vi "Parse Step Type.vi"(8 "error in (no error)":errorcluster, 9 "Sequence Context":refnum<class "Configuration.lvclass">, 10 "TestStand Result in":T2) -> (0 "error out":errorcluster, 2 "Step Type":T1=enum."String Value Test")   [LabVIEW 2020, in "Astemes_CSVReportPlugin.lvlib" / "TestStand Result Handler.lvclass"]
uses:
  TestStand Result Handler.lvclass
  Step Types.ctl
  Configuration/Configuration.lvclass
  TestStand Result.ctl
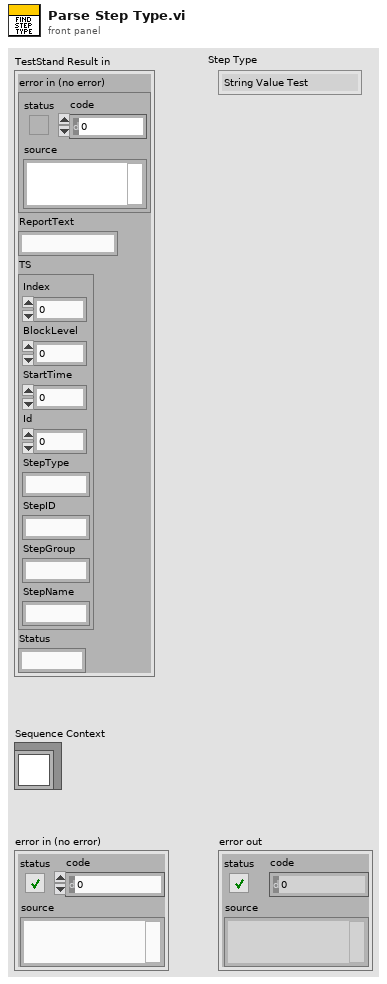
[diagram p1: front panel]
types:
  T1 = typedef "Astemes_CSVReportPlugin.lvlib/TestStand Result Handler.lvclass/Step Types.ctl" = enum16{"Unknown", "String Value Test", "Numeric Limit Test", "Action", "Flow Control"}
  T2 = typedef "Astemes_CSVReportPlugin.lvlib/TestStand Result Handler.lvclass/TestStand Result.ctl" = cluster{"error in (no error)":errorcluster, "ReportText":string, "TS":cluster{"Index":i32, "BlockLevel":i32, "StartTime":dbl, "Id":i32, "StepType":string, "StepID":string, "StepGroup":string, "StepName":string}, "Status":string}
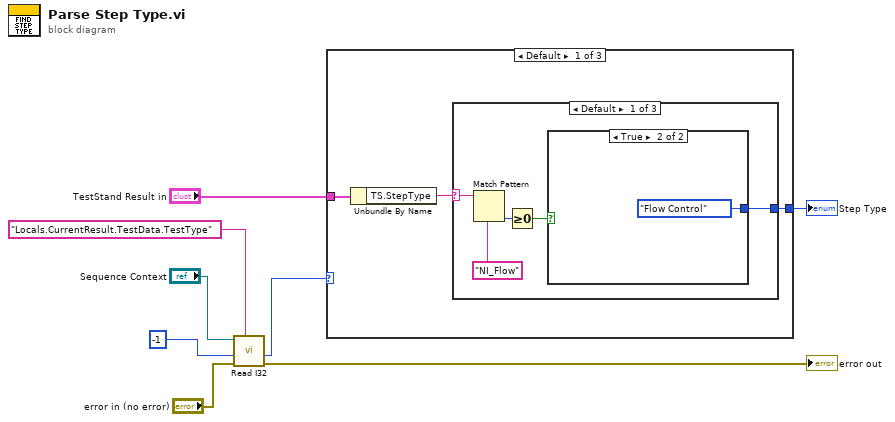
[diagram p0: block diagram]
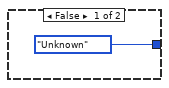
[diagram p2: hidden frame]
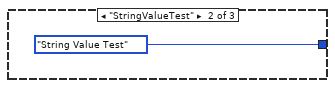
[diagram p3: hidden frame]
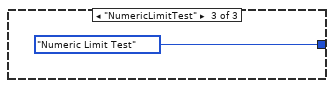
[diagram p4: hidden frame]
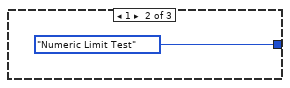
[diagram p5: hidden frame]
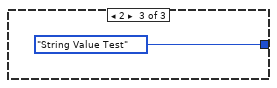
[diagram p6: hidden frame]
diagram:
  n1 = call-dynamic "Read I32.vi"("key"="Locals.CurrentResult.TestData.TestType", "error in (no error)"="error in (no error)", "default value"=-1, "Configuration In"="Sequence Context") -> ("error out"=→"error out":errorcluster, "value"=w2:i32)  [unwired: 5 in, 1 out]
  n2 = case shown="Default" w2 {
    tunnel: "TestStand Result in" -> [w11 _ _]
    tunnel: [w9 Step_Types."Numeric Limit Test" ("Step Type") Step_Types."String Value Test" ("Step Type")] -> w6
    frame Default {
      n3 = Unbundle By Name(w11) -> ("TS.StepType"=w10:string)
      n4 = case shown="Default" w10 {
        selector: w10 -> [w15 _ _]
        tunnel: [w16 Step_Types."String Value Test" ("Step Type") Step_Types."Numeric Limit Test" ("Step Type")] -> w9
        frame Default {
          n5 = Match Pattern(string=w15, regular expression="NI_Flow") -> (offset past match=w13:i32)  [unwired: 1 in, 3 out]
          n6 = Greater Or Equal To 0?(x=w13) -> (x >= 0?=w12:bool)
          n7 = case shown="True" w12 {
            tunnel: [Step_Types."Unknown" ("Step Type") Step_Types."Flow Control" ("Step Type")] -> w16
            frame False {
            }
            frame True {
            }
          }
        }
        frame "StringValueTest" {
        }
        frame "NumericLimitTest" {
        }
      }
    }
    frame 1 {
    }
    frame 2 {
    }
  }
  "Step Type" <- w6
